vi "Define Default Prefix.vi"(8 "error in":errorcluster, 11 "PWM output channel in":refnum<class "PWM Output Channel.lvclass">) -> (0 "error out":errorcluster, 3 "PWM output channel out":refnum<class "PWM Output Channel.lvclass">)   [LabVIEW 2020, in "Scan Engine Scripting.lvlib" / "PWM Output Channel.lvclass"]
uses:
  PWM Output Channel.lvclass
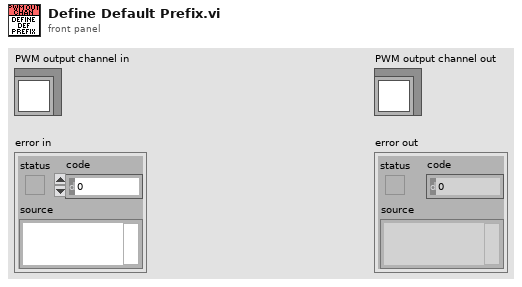
[diagram p1: front panel]
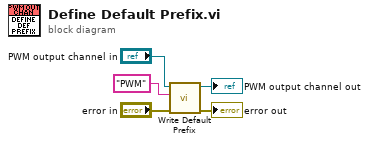
[diagram p0: block diagram]
diagram:
  n1 = call-dynamic "Write Default Prefix.vi"("error in"="error in", "default prefix"="PWM", "channel in"="PWM output channel in") -> ("error out"=→"error out":errorcluster, "channel out"=→"PWM output channel out":refnum<class "PWM Output Channel.lvclass">)  [unwired: 7 in]
